vi "Main_v2.vi"() -> ()   [LabVIEW 2020]
uses:
  Shutter-DQMH/Libraries/Shutter/Shutter State.ctl
  <vilib>/Analysis/1siggen.llb/Ramp Pattern by Delta.vi
  SMC100-DQMH/Libraries/SMC100/SMC100.lvlib
  <vilib>/Analysis/NI_AALBase.lvlib
  Shutter-DQMH/Libraries/Shutter/Shutter.lvlib
panel:
  in  "CLOSED Shutter Time (s)":dbl=6.0
  in  "Fine?":bool=TRUE
  in  "Fine Steps":dbl=0.01 format="%#_6f"
  in  "Fine End":dbl=10.7
  in  "Fine Start":dbl=10.6
  out "Position":dbl=10.2
  out "Shutter State":bool
  in  "Open Shutter Panel":bool
  in  "Open Delay Stage Panel":bool
  in  "SMC100 Serial Port":u8=3
  in  "Run":bool
  out "Seconds Running":i16
  in  "OPEN Shutter Time (s)":dbl=3.0
  out "Number of Steps":i32=20
  in  "Step Size":dbl=0.09999999999999998 format="%#_6f"
  in  "End Position":dbl=11.0
  in  "Start Position":dbl=10.0
  in  "Exit":bool
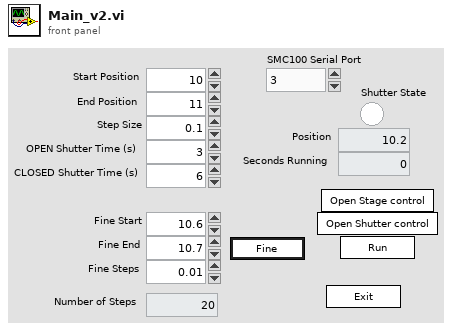
[diagram p1: front panel]
types:
  T1 = enum32{"Invalid", "Standard", "Closed", "Hidden", "Minimized", "Maximized"}
  T2 = enum32{"invalid app kind", "Development System", "Run Time System", "Student Edition", "Embedded LabVIEW", "Evaluation", "Custom"}
  T3 = typedef "Shutter State.ctl" = enum16{"None", "Open", "Closed"}
  T4 = cluster{"Core":cluster{"Current VI Reference":refnum<vi>, "Close Panel on Exit?":bool}, "Delay Positions":dbl[], "OPEN Shutter Time (s)":dbl, "Position Index":i32, "CLOSED Shutter Time (s)":dbl}
  T5 = cluster{"Current VI Reference":refnum<vi>, "Close Panel on Exit?":bool}
  T6 = typedef "SMC100.lvlib/Get Abs Position (Reply Payload)--cluster.ctl" = cluster{"Absolute Position":dbl, "Get Abs Position_error":errorcluster}
  T7 = typedef "Shutter.lvlib/Get Shutter State (Reply Payload)--cluster.ctl" = cluster{"Shutter State":T3, "Get Shutter State_error":errorcluster}
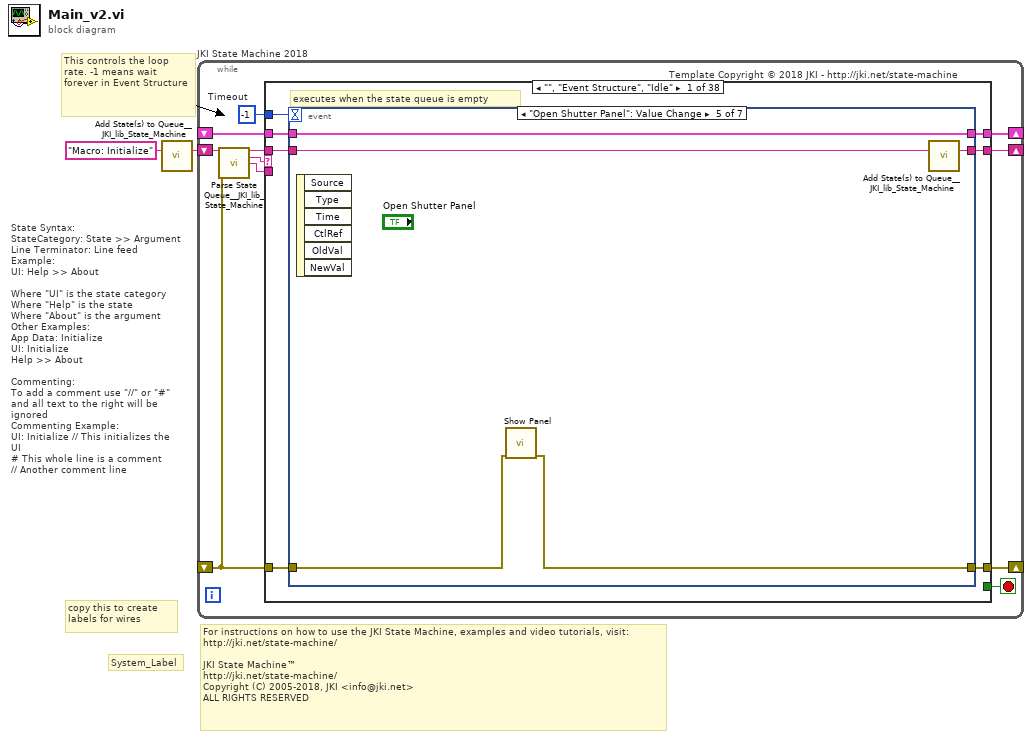
[diagram p0: block diagram]
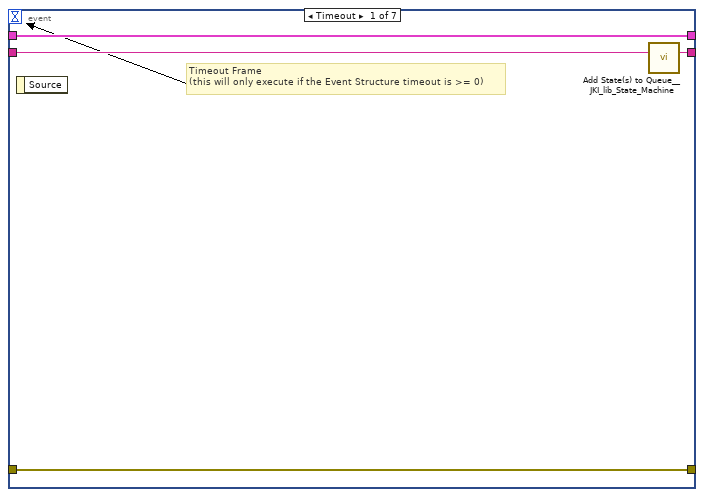
[diagram p2: hidden frame]
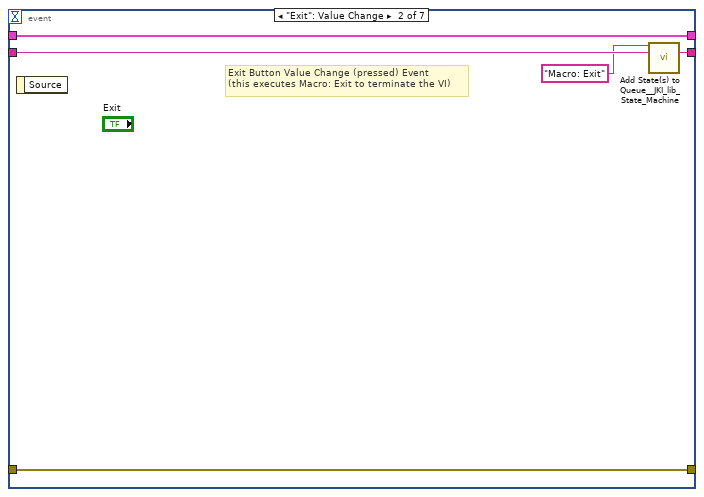
[diagram p3: hidden frame]
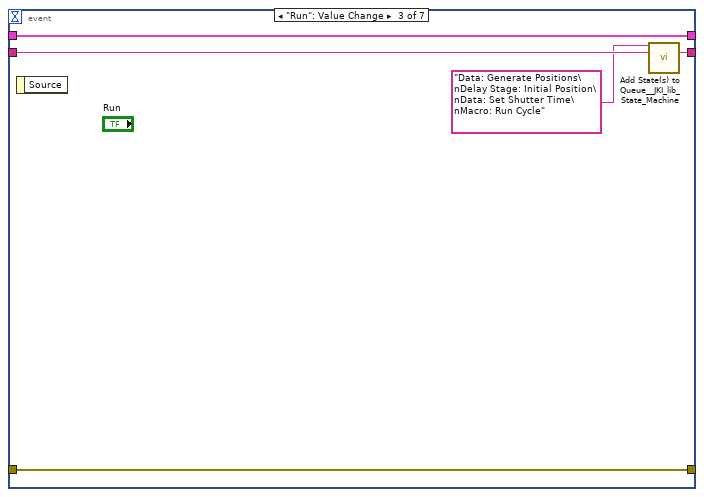
[diagram p4: hidden frame]
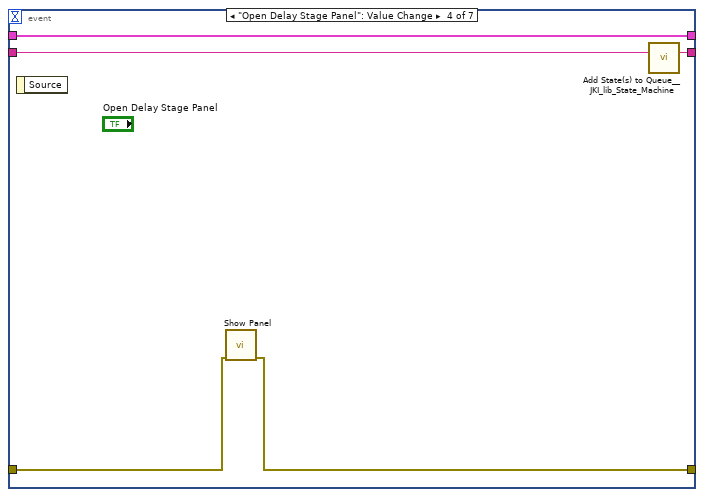
[diagram p5: hidden frame]
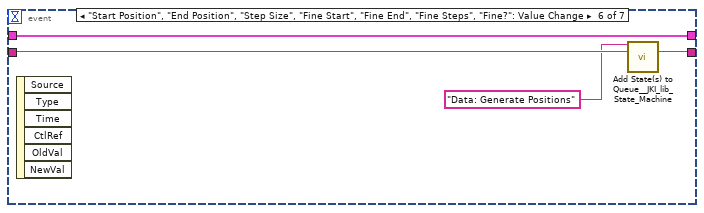
[diagram p6: hidden frame]
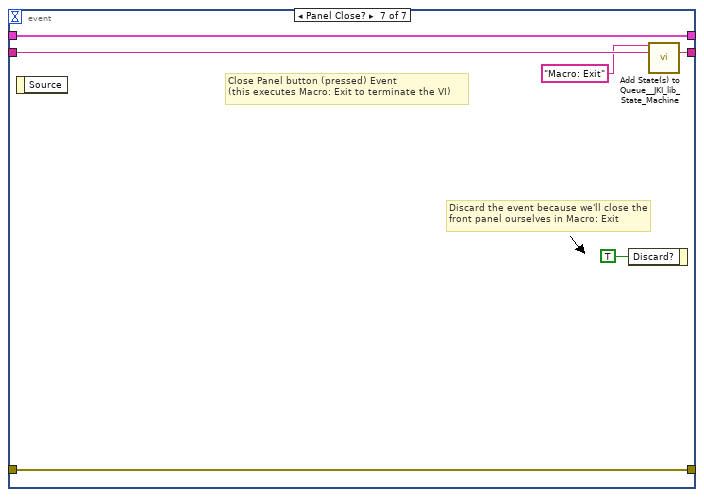
[diagram p7: hidden frame]
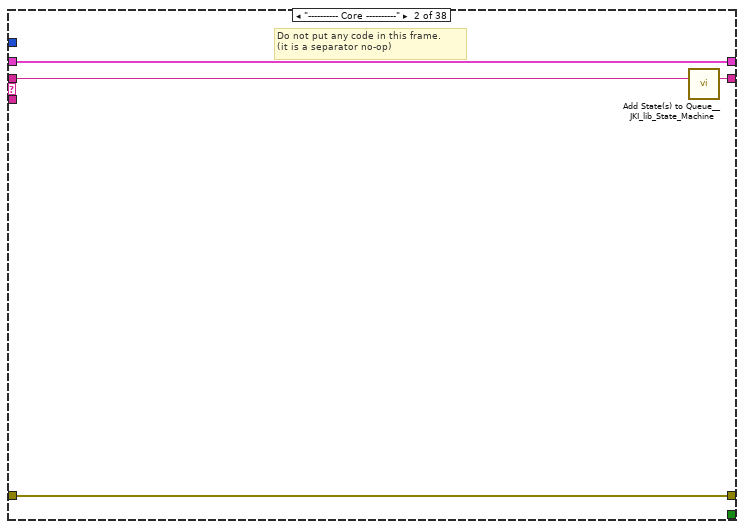
[diagram p8: hidden frame]
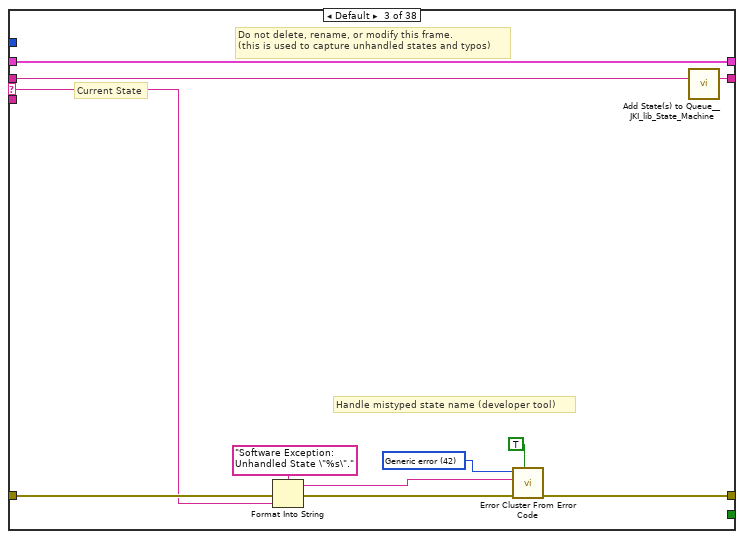
[diagram p9: hidden frame]
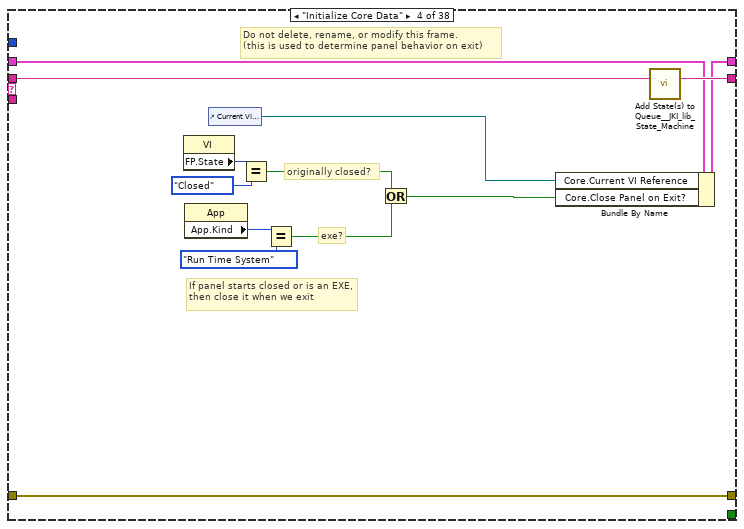
[diagram p10: hidden frame]
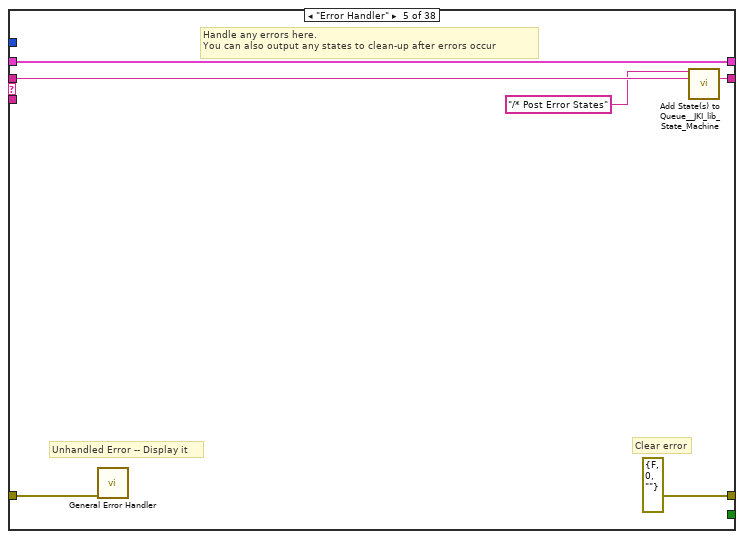
[diagram p11: hidden frame]
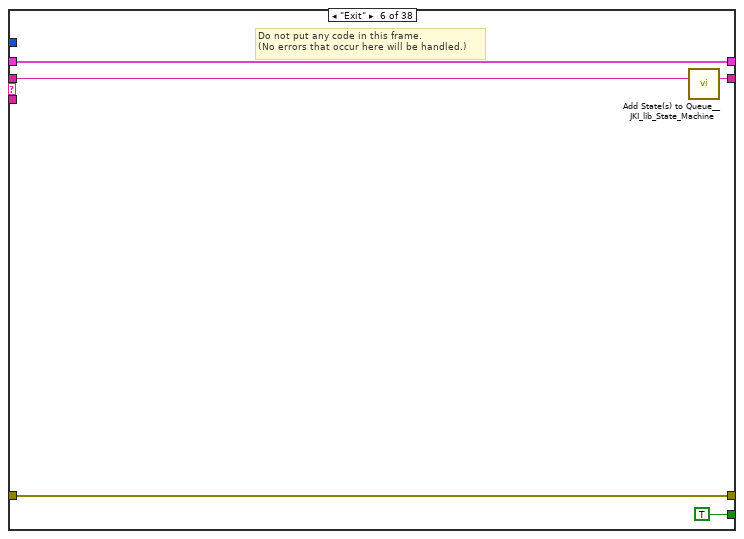
[diagram p12: hidden frame]
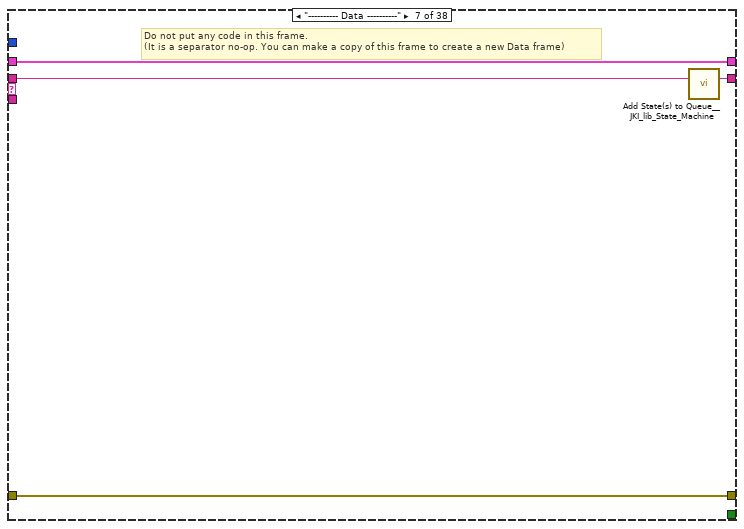
[diagram p13: hidden frame]
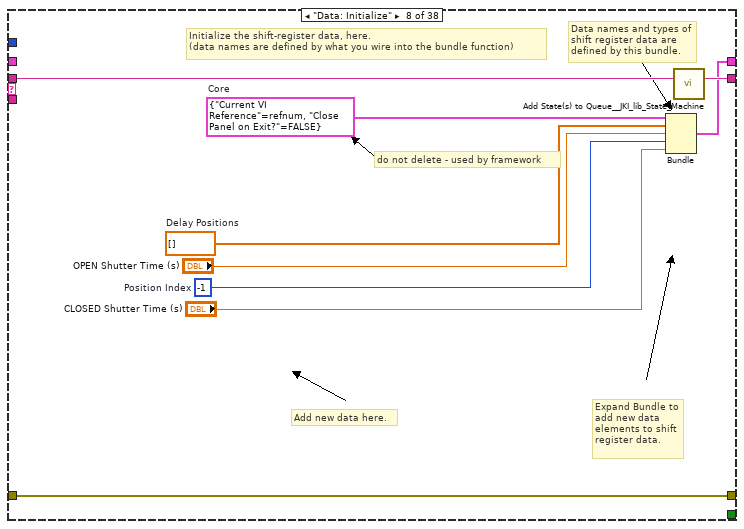
[diagram p14: hidden frame]
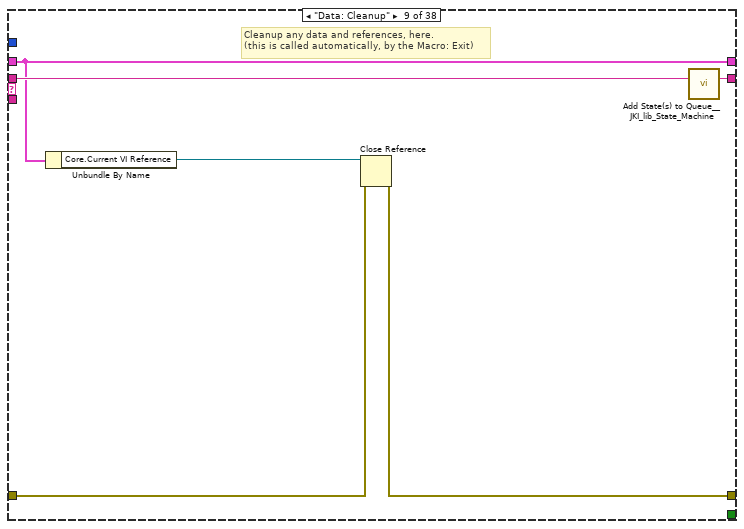
[diagram p15: hidden frame]
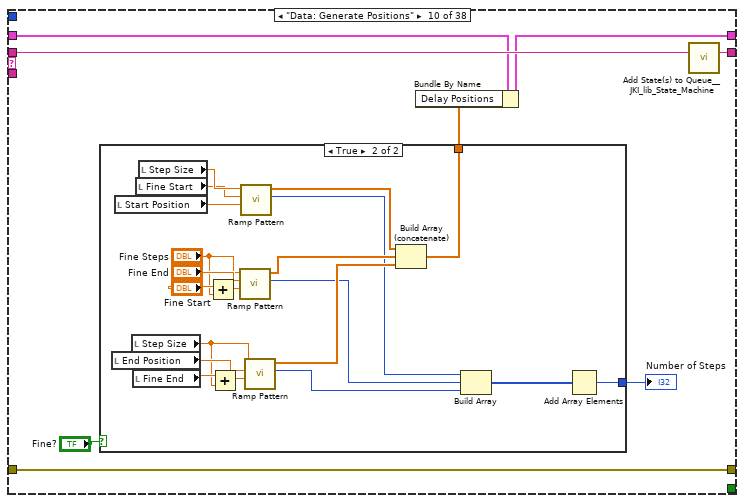
[diagram p16: hidden frame]
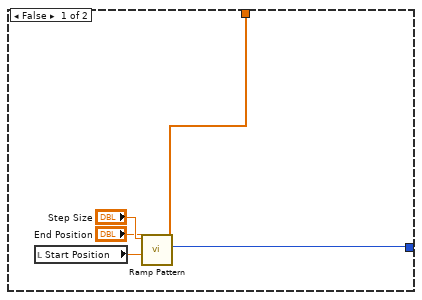
[diagram p17: hidden frame]
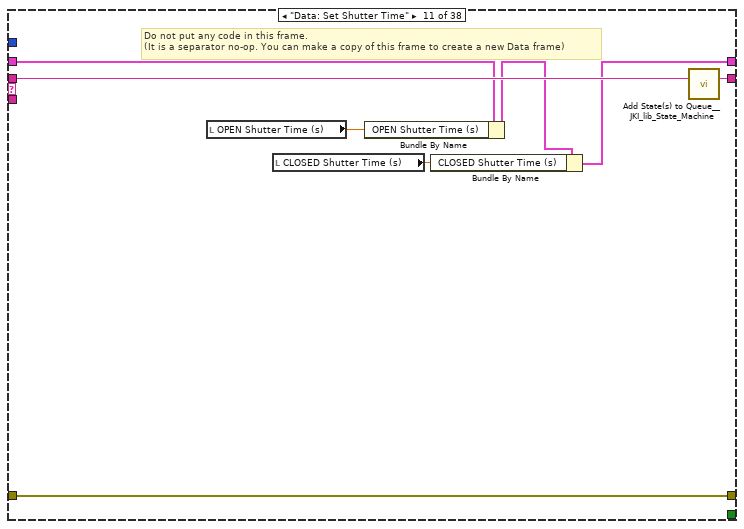
[diagram p18: hidden frame]
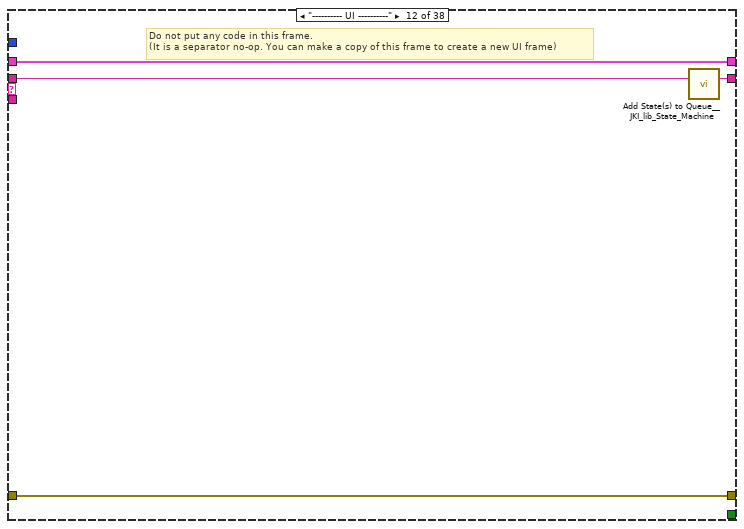
[diagram p19: hidden frame]
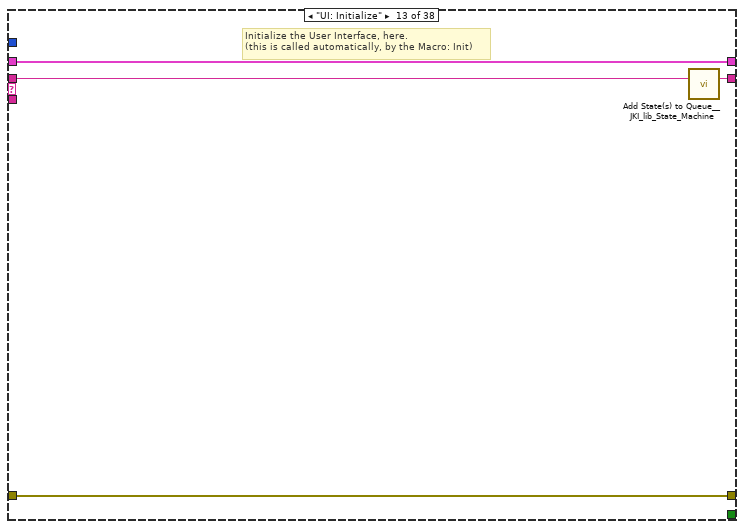
[diagram p20: hidden frame]
diagram:
  # "For instructions on how to use the JKI State Machine, examples and video tutorials, visit:\nhttp://jki.net/state-machine/\n\nJKI State Machine™\nhttp://jki.net/state-machine/\nCopyright (C) 2005-2018, JKI <info@jki.net>\nALL RIGHTS RESERVED"
  # "State Syntax:\nStateCategory: State >> Argument\nLine Terminator: Line feed\nExample:\nUI: Help >> About\n\nWhere \"UI\" is the state category\nWhere \"Help\" is the state\nWhere \"About\" is the argument\nOther Examples:\nApp Data: Initialize\nUI: Initialize\nHelp >> About\n\nCommenting:\nTo add a comment use \"//\" or \"#\" and all text to the right will be ignored\nCommenting Example:\nUI: Initialize // This initializes the UI\n# This whole line is a comment\n// Another comment line"
  # "copy this to create labels for wires"
  # "This controls the loop rate. -1 means wait forever in Event Structure"
  # "System_Label"
  n1 = call <vilib>:"Add State(s) to Queue__JKI_lib_State_Machine.vi"("State(s) in (\"\")"="Macro: Initialize") -> ("States Out"=w2:string)  [unwired: 14 in]
  n2 = while "JKI State Machine 2018" {
    shift-right: [w6] -> _
    shift-left: _ -> [w5]
    shift-right: [w9] -> _
    shift-left: _ -> [w3]
    shift-right: [w8] -> _
    shift-left: w2 -> [w10]
    stop <- w7 stop-if-true
    w4 = -1  # Timeout
    # "Template Copyright © 2018 JKI - http://jki.net/state-machine"
    n3 = call <vilib>:"Parse State Queue__JKI_lib_State_Machine.vi"("State Queue"=w10, "Error In (no error)"=w3) -> ("Remaining States"=w12:string, "Current State"=w13:string, "Arguments"=w11:string)  [unwired: 11 in]
    n4 = case shown="\"\", \"Event Structure\", \"Idle\"" w13 {
      selector: w13 -> [_ _ w59 _ _ _ _ _ _ _ _ _ _ _ _ _ _ _ _ _ _ _ _ _ _ _ _ _ _ _ _ _ _ _ _ _ _ _]
      tunnel: w12 -> [w20 w58 w63 w82 w88 w93 w97 w106 w112 w120 w153 w157 w161 w167 w178 w246 w252 w257 w262 w267 w277 w282 w286 w292 w297 w303 w314 w321 w325 w330 w335 w342 w349 w358 w362 w377 w387 w402]
      tunnel: w11 -> [_ _ _ _ _ _ _ _ _ _ _ _ _ w162 w172 _ _ _ _ _ _ _ _ _ _ _ _ _ _ _ _ _ _ _ _ _ _ _]
      tunnel: w5 -> [w18 w55 w61 w75 w85 w91 w94 _ w107 w117 w150 w154 w159 w165 w174 w245 w249 w254 w259 w264 w274 w279 w283 w289 w294 w300 w310 w318 w322 w327 w332 w339 w346 w356 w359 w374 w383 w398]
      tunnel: [w17 w56 w65 w79 errorcluster {"status"=FALSE, "code"=0, "source"=""} ("error out") w90 w95 w103 w108 w118 w151 w155 w158 w163 w175 w244 w250 w255 w260 w265 w275 w280 w284 w288 w293 w299 w311 w317 w323 w326 w331 w337 w345 w351 w360 w375 w385 w400] -> w9
      tunnel: w3 -> [w16 w56 w64 w79 w84 w90 w95 w103 w109 w118 w151 w155 w158 w164 w176 w244 w250 w255 w260 w265 w275 w280 w284 w290 w295 w301 w312 w319 w323 w328 w333 w340 w347 w352 w360 w375 w385 w400]
      tunnel: [w19 w57 w62 w81 w87 w92 w96 w105 w111 w119 w152 w156 w160 w166 w177 w247 w251 w256 w261 w266 w276 w281 w285 w291 w296 w302 w313 w320 w324 w329 w334 w341 w348 w357 w361 w376 w386 w401] -> w8
      tunnel: [_ _ _ _ _ TRUE _ _ _ _ _ _ _ _ _ _ _ _ _ _ _ _ _ _ _ _ _ _ _ _ _ _ _ _ _ _ _ _] -> w7
      tunnel: [w15 w55 w61 w80 w85 w91 w94 w104 w107 w116 w146 w154 w159 w165 w174 w245 w249 w254 w259 w264 w274 w279 w283 w289 w294 w300 w308 w318 w322 w327 w332 w339 w346 w356 w359 w370 w383 w398] -> w6
      tunnel: w4 -> [w14 _ _ _ _ _ _ _ _ _ _ _ _ _ _ _ _ _ _ _ _ _ _ _ _ _ _ _ _ _ _ _ _ _ _ _ _ _]
      frame "", "Event Structure", "Idle" {
        # "executes when the state queue is empty"
        n5 = event shown="[4] \"Open Shutter Panel\": Value Change" {
          selector: _ -> [_ _ _ _ _ _ _]
          dyn-events: _ -> [_ _ _ _ _ _ _]
          timeout: w14 -> [_ _ _ _ _ _ _]
          tunnel: w20 -> [w24 w29 w34 w39 w44 w46 w54]
          tunnel: [w23 w28 w33 w38 w43 w47 w53] -> w19
          tunnel: w18 -> [w21 w26 w31 w37 w42 w48 w51]
          tunnel: [w22 w27 w32 w36 w41 _ w52] -> w17
          tunnel: w16 -> [w22 w27 w32 w35 w40 _ w52]
          tunnel: [w21 w26 w31 w37 w42 w48 w51] -> w15
          event Timeout {
            # "Timeout Frame\n(this will only execute if the Event Structure timeout is >= 0)"
            n6 = event-data() -> ()  [unwired: 1 in, 1 out]
            n7 = call <vilib>:"Add State(s) to Queue__JKI_lib_State_Machine.vi"("State(s) in (\"\")"=w24) -> ("States Out"=w23:string)  [unwired: 14 in]
          }
          event "Exit": Value Change {
            # "Exit Button Value Change (pressed) Event\n(this executes Macro: Exit to terminate the VI)"
            n8 = event-data() -> ()  [unwired: 1 in, 1 out]
            n9 = call <vilib>:"Add State(s) to Queue__JKI_lib_State_Machine.vi"("State(s) in Front (\"\")"="Macro: Exit", "State(s) in (\"\")"=w29) -> ("States Out"=w28:string)  [unwired: 13 in]
          }
          event "Run": Value Change {
            n10 = event-data() -> ()  [unwired: 1 in, 1 out]
            n11 = call <vilib>:"Add State(s) to Queue__JKI_lib_State_Machine.vi"("State(s) in Front (\"\")"="Data: Generate Positions\nDelay Stage: Initial Position\nData: Set Shutter Time\nMacro: Run Cycle", "State(s) in (\"\")"=w34) -> ("States Out"=w33:string)  [unwired: 13 in]
          }
          event "Open Delay Stage Panel": Value Change {
            n12 = event-data() -> ()  [unwired: 1 in, 1 out]
            n13 = call "Show Panel.vi"("error in (no error)"=w35) -> ("error out"=w36:errorcluster)  [unwired: 10 in]
            n14 = call <vilib>:"Add State(s) to Queue__JKI_lib_State_Machine.vi"("State(s) in (\"\")"=w39) -> ("States Out"=w38:string)  [unwired: 14 in]
          }
          event "Open Shutter Panel": Value Change {
            n15 = event-data() -> ()  [unwired: 1 in, 6 out]
            n16 = call "Show Panel.vi"("error in (no error)"=w40) -> ("error out"=w41:errorcluster)  [unwired: 10 in]
            n17 = call <vilib>:"Add State(s) to Queue__JKI_lib_State_Machine.vi"("State(s) in (\"\")"=w44) -> ("States Out"=w43:string)  [unwired: 14 in]
          }
          event "Start Position", "End Position", "Step Size", "Fine Start", "Fine End", "Fine Steps", "Fine?": Value Change {
            n18 = event-data() -> ()  [unwired: 1 in, 6 out]
            n19 = call <vilib>:"Add State(s) to Queue__JKI_lib_State_Machine.vi"("State(s) in Front (\"\")"="Data: Generate Positions" ("State(s) in Front (\"\")"), "State(s) in (\"\")"=w46) -> ("States Out"=w47:string)  [unwired: 13 in]
          }
          event Panel Close? {
            # "Discard the event because we'll close the front panel ourselves in Macro: Exit"
            # "Close Panel button (pressed) Event\n(this executes Macro: Exit to terminate the VI)"
            n20 = event-data() -> ()  [unwired: 1 in, 1 out]
            n21 = event-data("Discard?"=TRUE) -> ()  [unwired: 1 in, 1 out]
            n22 = call <vilib>:"Add State(s) to Queue__JKI_lib_State_Machine.vi"("State(s) in Front (\"\")"="Macro: Exit", "State(s) in (\"\")"=w54) -> ("States Out"=w53:string)  [unwired: 13 in]
          }
        }
      }
      frame "---------- Core ----------" {
        # "Do not put any code in this frame.\n(it is a separator no-op)"
        n23 = call <vilib>:"Add State(s) to Queue__JKI_lib_State_Machine.vi"("State(s) in (\"\")"=w58) -> ("States Out"=w57:string)  [unwired: 14 in]
      }
      frame Default {
        w68 = 42 items=["No error", "Argument error", "Memory is full", "Out of zone", "End of file", "File already open", "Generic file I/O error", "File not found", "File permission error", "Disk is full", "Duplicate path", "Too many files open", "System feature not enabled", "Resource file not found", "Cannot add resource", "Resource not found", "Image not found", "Image memory error", "Pen does not exist", "Config type invalid", "Config token not found", "Config parse error", "Config memory error", "Bad external code format", "Bad external code offset", "External code not present", "Null window", "Destroy window error", "Null menu", "Print aborted", "Bad print record", "Print driver error", "Windows error during printing", "Memory error during printing", "Print dialog error", "Generic print error", "Invalid device refnum", "Device not found", "Device parameter error", "Device unit error", "Cannot open device", "Device call aborted", "Generic error", "Cancelled by user", "Object ID too low", "Object ID too high", "Object not in heap", "Unknown heap", "Unknown object (invalid DefProc)", "Unknown object (DefProc not in table)", "Message out of range", "Invalid (null) method", "Unknown message", "Manager call not supported", "Bad address", "Network operation in progress", "Network operation timed out", "Connection is busy", "Network attribute not supported", "Network error", "Address in use", "System out of memory", "Connection aborted", "Connection refused", "Not connected", "Already connected", "Connection closed", "Initialization error (interapplication manager)", "Bad occurrence", "Wait on unbound occurrence handler", "Occurrence queue overflow", "Datalog type conflict", "Unused", "Unrecognized type (interapplication manager)", "Memory corrupt", "Failed to make temporary DLL", "Old CIN version", "Drag socket not found", "Failed to load drop-object", "Failed to register OLE object", "Failed to release OLE object", "Format specifier type mismatch", "Unknown format specifier", "Too few format specifiers", "Too many format specifiers", "Scan failed", "Newer CIN version", "Error converting to variant", "Runtime menu error", "Password tampered", "Variant attribute not found", "Incompatible variant data type", "Event data is not available", "Event Store is not present", "Occurrence is not found", "Event Queue is not created", "Event info is not available", "Refnum passed is NULL", "Error retrieving Class GUID", "Error retrieving CoClass GUID", "Error retrieving TypeLib GUID.", "Bad built application magic bytes.", "Specific driver is different from the specific driver associated with the Logical Name.", "There is no session opened to the class driver.", "Max Error", "MAX - Error with config objects", "MAX - Error loading configuration", "MAX - Group not supported"]
        # "Current State"
        # "Do not delete, rename, or modify this frame.\n(this is used to capture unhandled states and typos)"
        # "Handle mistyped state name (developer tool)"
        n24 = Format Into String(format string="Software Exception: Unhandled State \"%s\"." ("message"), error in=w64, w59) -> (resulting string=w67:string, error out=w66:errorcluster)  [unwired: 1 in]
        n25 = call <vilib>:"Error Cluster From Error Code.vi"("show call chain? (False)"=TRUE, "error in (no error)"=w66, "error message (\"\")"=w67, "error code (0)"=w68) -> ("error out"=w65:errorcluster)  [unwired: 5 in]
        n26 = call <vilib>:"Add State(s) to Queue__JKI_lib_State_Machine.vi"("State(s) in (\"\")"=w63) -> ("States Out"=w62:string)  [unwired: 14 in]
      }
      frame "Initialize Core Data" {
        # "Do not delete, rename, or modify this frame.\n(this is used to determine panel behavior on exit)"
        # "originally closed?"
        # "exe?"
        # "If panel starts closed or is an EXE, then close it when we exit"
        n27 = property class="VI"() -> ("FP.State"=w72:T1)  [unwired: 2 in, 2 out]
        n28 = property class="App"() -> ("App.Kind"=w78:T2)  [unwired: 2 in, 2 out]
        n29 = control-ref of="Current VI Reference"() -> (w73:refnum<vi>)
        n30 = Equal?(x=w72, y=T1."Closed" ("Front Panel Window:State")) -> (x = y?=w70:bool)
        n31 = Equal?(x=w78, y=T2."Run Time System" ("Application:Kind")) -> (x = y?=w76:bool)
        n32 = Or(x=w70, y=w76) -> (x .or. y?=w74:bool)
        n33 = Bundle By Name(cluster=w75, "Core.Current VI Reference"=w73, "Core.Close Panel on Exit?"=w74) -> (w80:T4)
        n34 = call <vilib>:"Add State(s) to Queue__JKI_lib_State_Machine.vi"("State(s) in (\"\")"=w82) -> ("States Out"=w81:string)  [unwired: 14 in]
      }
      frame "Error Handler" {
        # "Unhandled Error -- Display it"
        # "Handle any errors here.\nYou can also output any states to clean-up after errors occur"
        # "Clear error"
        n35 = call <vilib>:"General Error Handler.vi"("error in (no error)"=w84) -> ()  [unwired: 10 in, 5 out]
        n36 = call <vilib>:"Add State(s) to Queue__JKI_lib_State_Machine.vi"("State(s) in Front (\"\")"="/* Post Error States", "State(s) in (\"\")"=w88) -> ("States Out"=w87:string)  [unwired: 13 in]
      }
      frame "Exit" {
        # "Do not put any code in this frame.\n(No errors that occur here will be handled.)"
        n37 = call <vilib>:"Add State(s) to Queue__JKI_lib_State_Machine.vi"("State(s) in (\"\")"=w93) -> ("States Out"=w92:string)  [unwired: 14 in]
      }
      frame "---------- Data ----------" {
        # "Do not put any code in this frame.\n(It is a separator no-op. You can make a copy of this frame to create a new Data frame)"
        n38 = call <vilib>:"Add State(s) to Queue__JKI_lib_State_Machine.vi"("State(s) in (\"\")"=w97) -> ("States Out"=w96:string)  [unwired: 14 in]
      }
      frame "Data: Initialize" {
        w100 = -1  # Position Index
        w101 = dbl[] []  # Delay Positions
        w102 = T5 {"Current VI Reference"=refnum, "Close Panel on Exit?"=FALSE}  # Core
        # "do not delete - used by framework"
        # "Expand Bundle to add new data elements to shift register data."
        # "Add new data here."
        # "Data names and types of shift register data are defined by this bundle."
        # "Initialize the shift-register data, here.\n(data names are defined by what you wire into the bundle function)"
        n39 = Bundle("Core"=w102, "Delay Positions"=w101, "OPEN Shutter Time (s)"="OPEN Shutter Time (s)", "Position Index"=w100, "CLOSED Shutter Time (s)"="CLOSED Shutter Time (s)") -> (w104:T4)  [unwired: 1 in]
        n40 = call <vilib>:"Add State(s) to Queue__JKI_lib_State_Machine.vi"("State(s) in (\"\")"=w106) -> ("States Out"=w105:string)  [unwired: 14 in]
      }
      frame "Data: Cleanup" {
        # "Cleanup any data and references, here.\n(this is called automatically, by the Macro: Exit)"
        n41 = Unbundle By Name(w107) -> ("Core.Current VI Reference"=w110:refnum<vi>)
        n42 = Close Reference(reference=w110, error in (no error)=w109) -> (error out=w108:errorcluster)
        n43 = call <vilib>:"Add State(s) to Queue__JKI_lib_State_Machine.vi"("State(s) in (\"\")"=w112) -> ("States Out"=w111:string)  [unwired: 14 in]
      }
      frame "Data: Generate Positions" {
        n44 = case shown="True" "Fine?" {
          tunnel: [w122 w127] -> w114
          tunnel: [w121 w126] -> w113
          frame False {
            n45 = local read "Start Position"() -> (w123:dbl)
            n46 = call-poly <vilib>:"Ramp Pattern.vi"("start"=w123, "end"="End Position", "delta"="Step Size") -> ("samples"=w122:i32, "Ramp Pattern"=w121:dbl[])  [unwired: 6 in, 1 out]
          }
          frame True {
            n47 = local read "End Position"() -> (w138:dbl)
            n48 = local read "Start Position"() -> (w143:dbl)
            n49 = local read "Step Size"() -> (w135:dbl)
            n50 = local read "Fine End"() -> (w137:dbl)
            n51 = local read "Fine Start"() -> (w141:dbl)
            n52 = local read "Step Size"() -> (w142:dbl)
            n53 = Add(x="Fine Start", y="Fine Steps") -> (x+y=w140:dbl)
            n54 = Add(x=w137, y=w135) -> (x+y=w136:dbl)
            n55 = call-poly <vilib>:"Ramp Pattern.vi"("start"=w140, "end"="Fine End", "delta"="Fine Steps") -> ("samples"=w130:i32, "Ramp Pattern"=w133:dbl[])  [unwired: 6 in, 1 out]
            n56 = call-poly <vilib>:"Ramp Pattern.vi"("start"=w143, "end"=w141, "delta"=w142) -> ("samples"=w129:i32, "Ramp Pattern"=w134:dbl[])  [unwired: 6 in, 1 out]
            n57 = call-poly <vilib>:"Ramp Pattern.vi"("start"=w136, "end"=w138, "delta"=w135) -> ("samples"=w131:i32, "Ramp Pattern"=w132:dbl[])  [unwired: 6 in, 1 out]
            n58 = Build Array (concatenate)(w134, w133, w132) -> (w126:dbl[])
            n59 = Build Array(w129, w130, w131) -> (w128:i32[])
            n60 = Add Array Elements(numeric array=w128) -> (sum=w127:i32)
          }
        }
        "Number of Steps" <- w114
        n61 = Bundle By Name(cluster=w117, "Delay Positions"=w113) -> (w116:T4)
        n62 = call <vilib>:"Add State(s) to Queue__JKI_lib_State_Machine.vi"("State(s) in (\"\")"=w120) -> ("States Out"=w119:string)  [unwired: 14 in]
      }
      frame "Data: Set Shutter Time" {
        # "Do not put any code in this frame.\n(It is a separator no-op. You can make a copy of this frame to create a new Data frame)"
        n63 = local read "OPEN Shutter Time (s)"() -> (w149:dbl)
        n64 = local read "CLOSED Shutter Time (s)"() -> (w148:dbl)
        n65 = Bundle By Name(cluster=w150, "OPEN Shutter Time (s)"=w149) -> (w147:T4)
        n66 = Bundle By Name(cluster=w147, "CLOSED Shutter Time (s)"=w148) -> (w146:T4)
        n67 = call <vilib>:"Add State(s) to Queue__JKI_lib_State_Machine.vi"("State(s) in (\"\")"=w153) -> ("States Out"=w152:string)  [unwired: 14 in]
      }
      frame "---------- UI ----------" {
        # "Do not put any code in this frame.\n(It is a separator no-op. You can make a copy of this frame to create a new UI frame)"
        n68 = call <vilib>:"Add State(s) to Queue__JKI_lib_State_Machine.vi"("State(s) in (\"\")"=w157) -> ("States Out"=w156:string)  [unwired: 14 in]
      }
      frame "UI: Initialize" {
        # "Initialize the User Interface, here.\n(this is called automatically, by the Macro: Init)"
        n69 = call <vilib>:"Add State(s) to Queue__JKI_lib_State_Machine.vi"("State(s) in (\"\")"=w161) -> ("States Out"=w160:string)  [unwired: 14 in]
      }
      frame "UI: Cursor Set" {
        # "Argument"
        # "Set and Unset Cursor Busy.\n(Usage: \"UI: Cursor Set >> Busy|Idle\")"
        n70 = case shown="\"Idle\", Default" w162 {
          tunnel: w164 -> [w169 w171]
          tunnel: [w168 w170] -> w163
          frame "Idle", Default {
            n71 = call <vilib>:"Unset Busy.vi"("error in (no error)"=w169) -> ("error out"=w168:errorcluster)  [unwired: 10 in]
          }
          frame "Busy" {
            n72 = call <vilib>:"Set Busy.vi"("error in (no error)"=w171) -> ("error out"=w170:errorcluster)  [unwired: 9 in, 1 out]
          }
        }
        n73 = call <vilib>:"Add State(s) to Queue__JKI_lib_State_Machine.vi"("State(s) in (\"\")"=w167) -> ("States Out"=w166:string)  [unwired: 14 in]
      }
      frame "UI: Front Panel State" {
        # "Argument"
        # "Set Front Panel Open or Closed\n(Usage: \"UI: Front Panel State >> Open|Close\")"
        n74 = Unbundle By Name(w174) -> ("Core.Current VI Reference"=w173:refnum<vi>)
        n75 = case shown="\"Minimize\", \"Minimized\"" w172 {
          tunnel: w176 -> [w184 w199 w210 w223 w236]
          tunnel: [w186 w200 w212 w225 w238] -> w175
          tunnel: w173 -> [w185 w197 w211 w224 w237]
          frame "Open", "Standard", Default {
            w179 = T1."Standard" ("State")
            n76 = property class="VI"(reference=w185, error in=w184) -> (reference out=w182:refnum<vi>, error out=w183:errorcluster, "FP.State"=w181:T1)
            n77 = Not Equal?(x=w181, y=w179) -> (x != y?=w180:bool)
            n78 = case shown="True" w180 {
              tunnel: [w190 w192] -> w186
              tunnel: w183 -> [w189 w192]
              tunnel: w182 -> [w188 _]
              tunnel: w179 -> [w187 _]
              frame True {
                n79 = invoke class="VI" method="FP.Open"(reference=w188, error in=w189, "Activate"=TRUE, "State"=w187) -> (error out=w190:errorcluster)  [unwired: 1 in, 4 out]
              }
              frame False {
              }
            }
          }
          frame "Close", "Closed" {
            n80 = property class="VI"(reference=w197, error in=w199) -> (reference out=w196:refnum<vi>, error out=w198:errorcluster, "FP.State"=w194:T1)
            n81 = Not Equal?(x=w194, y=T1."Closed" ("Front Panel Window:State")) -> (x != y?=w193:bool)
            n82 = case shown="True" w193 {
              tunnel: [w201 w204] -> w200
              tunnel: w198 -> [w201 w203]
              tunnel: w196 -> [_ w202]
              frame False {
              }
              frame True {
                n83 = invoke class="VI" method="FP.Close"(reference=w202, error in=w203) -> (error out=w204:errorcluster)  [unwired: 1 in, 2 out]
              }
            }
          }
          frame "Hidden", "Hide" {
            w205 = T1."Hidden" ("State")
            n84 = property class="VI"(reference=w211, error in=w210) -> (reference out=w208:refnum<vi>, error out=w209:errorcluster, "FP.State"=w207:T1)
            n85 = Not Equal?(x=w207, y=w205) -> (x != y?=w206:bool)
            n86 = case shown="True" w206 {
              tunnel: [w216 w217] -> w212
              tunnel: w209 -> [w215 w217]
              tunnel: w208 -> [w214 _]
              tunnel: w205 -> [w213 _]
              frame True {
                n87 = invoke class="VI" method="FP.Open"(reference=w214, error in=w215, "State"=w213) -> (error out=w216:errorcluster)  [unwired: 2 in, 4 out]
              }
              frame False {
              }
            }
          }
          frame "Minimize", "Minimized" {
            w218 = T1."Minimized" ("State")
            n88 = property class="VI"(reference=w224, error in=w223) -> (reference out=w221:refnum<vi>, error out=w222:errorcluster, "FP.State"=w220:T1)
            n89 = Not Equal?(x=w220, y=w218) -> (x != y?=w219:bool)
            n90 = case shown="True" w219 {
              tunnel: [w229 w230] -> w225
              tunnel: w222 -> [w228 w230]
              tunnel: w221 -> [w227 _]
              tunnel: w218 -> [w226 _]
              frame True {
                n91 = invoke class="VI" method="FP.Open"(reference=w227, error in=w228, "State"=w226) -> (error out=w229:errorcluster)  [unwired: 2 in, 4 out]
              }
              frame False {
              }
            }
          }
          frame "Maximize", "Maximized" {
            w231 = T1."Maximized" ("State")
            n92 = property class="VI"(reference=w237, error in=w236) -> (reference out=w234:refnum<vi>, error out=w235:errorcluster, "FP.State"=w233:T1)
            n93 = Not Equal?(x=w233, y=w231) -> (x != y?=w232:bool)
            n94 = case shown="True" w232 {
              tunnel: [w242 w243] -> w238
              tunnel: w235 -> [w241 w243]
              tunnel: w234 -> [w240 _]
              tunnel: w231 -> [w239 _]
              frame True {
                n95 = invoke class="VI" method="FP.Open"(reference=w240, error in=w241, "State"=w239) -> (error out=w242:errorcluster)  [unwired: 2 in, 4 out]
              }
              frame False {
              }
            }
          }
        }
        n96 = call <vilib>:"Add State(s) to Queue__JKI_lib_State_Machine.vi"("State(s) in (\"\")"=w178) -> ("States Out"=w177:string)  [unwired: 14 in]
      }
      frame "UI: Stop Exit" {
        n97 = local write "Exit"(FALSE ("Run")) -> ()
        n98 = call <vilib>:"Add State(s) to Queue__JKI_lib_State_Machine.vi"("State(s) in (\"\")"=w246) -> ("States Out"=w247:string)  [unwired: 14 in]
      }
      frame "---------- Macro ----------" {
        # "Do not put any code in this frame.\n(It is a separator no-op. You can make a copy of this frame to create a new Macro frame)"
        n99 = call <vilib>:"Add State(s) to Queue__JKI_lib_State_Machine.vi"("State(s) in (\"\")"=w252) -> ("States Out"=w251:string)  [unwired: 14 in]
      }
      frame "Macro: Run Cycle" {
        n100 = call <vilib>:"Add State(s) to Queue__JKI_lib_State_Machine.vi"("State(s) in Front (\"\")"="Shutter: Close\nShutter: Get Shutter State\nDelay Stage: Move Next\nDelay Stage: Get Position\nHelpers: Wait Closed\nShutter: Open\nShutter: Get Shutter State\nHelpers: Wait\nHelpers: At End?" ("State(s) in Front (\"\")"), "State(s) in (\"\")"=w257) -> ("States Out"=w256:string)  [unwired: 13 in]
      }
      frame "Macro: Initialize" {
        # "Initialization Macro\n(This is called once, when the VI starts)"
        n101 = call <vilib>:"Add State(s) to Queue__JKI_lib_State_Machine.vi"("State(s) in Front (\"\")"="Data: Initialize\nInitialize Core Data\nDelay Stage: Start Module\nShutter: Start Module\nUI: Initialize\nUI: Front Panel State >> Open\nUI: Stop Exit", "State(s) in (\"\")"=w262) -> ("States Out"=w261:string)  [unwired: 13 in]
      }
      frame "Macro: Initial Device States" {
        n102 = call <vilib>:"Add State(s) to Queue__JKI_lib_State_Machine.vi"("State(s) in Front (\"\")"="Delay Stage: Initial Position" ("State(s) in Front (\"\")"), "State(s) in (\"\")"=w267) -> ("States Out"=w266:string)  [unwired: 13 in]
      }
      frame "Macro: Exit" {
        # "Exit Macro\n(This is called once, when the VI exits)"
        n103 = Unbundle By Name(w274) -> ("Core.Close Panel on Exit?"=w273:bool)
        n104 = Select(t="UI: Front Panel State >> Close", s=w273, f="") -> (s? t:f=w270:string)
        n105 = call <vilib>:"Add State(s) to Queue__JKI_lib_State_Machine.vi"("State(s) in (\"\")"=w270, "State(s) at Back (\"\")"="Delay Stage: Stop Module\nShutter: Stop Module\nData: Cleanup\nExit") -> ("States Out"=w268:string)  [unwired: 13 in]
        n106 = call <vilib>:"Add State(s) to Queue__JKI_lib_State_Machine.vi"("State(s) in Front (\"\")"=w268, "State(s) in (\"\")"=w277) -> ("States Out"=w276:string)  [unwired: 13 in]
      }
      frame "Macro: Device Cleanup" {
        # "Do not put any code in this frame.\n(It is a separator no-op. You can make a copy of this frame to create a new Macro frame)"
        n107 = call <vilib>:"Add State(s) to Queue__JKI_lib_State_Machine.vi"("State(s) in Front (\"\")"="Shutter: Close\nShutter: Get Shutter State\nDelay Stage: Get Position\nUI: Stop Exit" ("State(s) in Front (\"\")"), "State(s) in (\"\")"=w282) -> ("States Out"=w281:string)  [unwired: 13 in]
      }
      frame "---------- Delay Stage ----------" {
        # "Template Separator\n(You can make a copy of, or modify, this frame)"
        n108 = call <vilib>:"Add State(s) to Queue__JKI_lib_State_Machine.vi"("State(s) in (\"\")"=w286) -> ("States Out"=w285:string)  [unwired: 14 in]
      }
      frame "Delay Stage: Start Module" {
        # "Template Separator\n(You can make a copy of, or modify, this frame)"
        n109 = call "Start Module.vi"("error in (no error)"=w290, "SerialPort"="SMC100 Serial Port") -> ("error out"=w288:errorcluster)  [unwired: 6 in, 3 out]
        n110 = call <vilib>:"Add State(s) to Queue__JKI_lib_State_Machine.vi"("State(s) in (\"\")"=w292) -> ("States Out"=w291:string)  [unwired: 14 in]
      }
      frame "Delay Stage: Stop Module" {
        # "Template Separator\n(You can make a copy of, or modify, this frame)"
        n111 = call "Stop Module.vi"("error in (no error)"=w295) -> ("error out"=w293:errorcluster)  [unwired: 10 in]
        n112 = call <vilib>:"Add State(s) to Queue__JKI_lib_State_Machine.vi"("State(s) in (\"\")"=w297) -> ("States Out"=w296:string)  [unwired: 14 in]
      }
      frame "Delay Stage: Initial Position" {
        # "Your code here.\n(You can make a copy of, or modify, this frame)"
        n113 = call "Set Abs Position.vi"("error in (no error)"=w301, "Abolute Position"="Start Position") -> ("error out"=w299:errorcluster)  [unwired: 9 in]
        n114 = call <vilib>:"Add State(s) to Queue__JKI_lib_State_Machine.vi"("State(s) in (\"\")"=w303) -> ("States Out"=w302:string)  [unwired: 14 in]
      }
      frame "Delay Stage: Move Next" {
        # "Your code here.\n(You can make a copy of, or modify, this frame)"
        n115 = Unbundle By Name(w310) -> ("Delay Positions"=w309:dbl[], "Position Index"=w307:i32)
        n116 = Increment(x=w307) -> (x+1=w306:i32)
        n117 = Bundle By Name(cluster=w310, "Position Index"=w306) -> (w308:T4)
        n118 = Index Array(array=w309, index=w306) -> (element=w305:dbl)
        n119 = call "Set Abs Position.vi"("error in (no error)"=w312, "Abolute Position"=w305) -> ("error out"=w311:errorcluster)  [unwired: 9 in]
        n120 = Wait (ms)(milliseconds to wait=u32 1000) -> ()  [unwired: 1 out]
        n121 = call <vilib>:"Add State(s) to Queue__JKI_lib_State_Machine.vi"("State(s) in (\"\")"=w314) -> ("States Out"=w313:string)  [unwired: 14 in]
      }
      frame "Delay Stage: Get Position" {
        # "Template Separator\n(You can make a copy of, or modify, this frame)"
        n122 = call "Get Abs Position.vi"("error in (no error)"=w319) -> ("error out"=w317:errorcluster, "Reply Payload"=w316:T6)  [unwired: 8 in, 1 out]
        n123 = Unbundle By Name(w316) -> ("Absolute Position"=→"Position":dbl)
        n124 = call <vilib>:"Add State(s) to Queue__JKI_lib_State_Machine.vi"("State(s) in (\"\")"=w321) -> ("States Out"=w320:string)  [unwired: 14 in]
      }
      frame "---------- Shutter ----------" {
        # "Your code here.\n(You can make a copy of, or modify, this frame)"
        n125 = call <vilib>:"Add State(s) to Queue__JKI_lib_State_Machine.vi"("State(s) in (\"\")"=w325) -> ("States Out"=w324:string)  [unwired: 14 in]
      }
      frame "Shutter: Start Module" {
        # "Your code here.\n(You can make a copy of, or modify, this frame)"
        n126 = call "Start Module.vi"("error in (no error)"=w328) -> ("error out"=w326:errorcluster)  [unwired: 7 in, 3 out]
        n127 = call <vilib>:"Add State(s) to Queue__JKI_lib_State_Machine.vi"("State(s) in (\"\")"=w330) -> ("States Out"=w329:string)  [unwired: 14 in]
      }
      frame "Shutter: Stop Module" {
        # "Your code here.\n(You can make a copy of, or modify, this frame)"
        n128 = call "Stop Module.vi"("error in (no error)"=w333) -> ("error out"=w331:errorcluster)  [unwired: 10 in]
        n129 = call <vilib>:"Add State(s) to Queue__JKI_lib_State_Machine.vi"("State(s) in (\"\")"=w335) -> ("States Out"=w334:string)  [unwired: 14 in]
      }
      frame "Shutter: Open" {
        # "Your code here.\n(You can make a copy of, or modify, this frame)"
        n130 = call "Set Shutter State.vi"("error in (no error)"=w340, "Shutter State"=Shutter_State."Open") -> ("error out"=w337:errorcluster)  [unwired: 7 in, 2 out]
        n131 = Wait (ms)(milliseconds to wait=u32 200) -> ()  [unwired: 1 out]
        n132 = call <vilib>:"Add State(s) to Queue__JKI_lib_State_Machine.vi"("State(s) in (\"\")"=w342) -> ("States Out"=w341:string)  [unwired: 14 in]
      }
      frame "Shutter: Close" {
        # "Your code here.\n(You can make a copy of, or modify, this frame)"
        n133 = call "Set Shutter State.vi"("error in (no error)"=w347, "Shutter State"=Shutter_State."Closed") -> ("error out"=w345:errorcluster)  [unwired: 7 in, 2 out]
        n134 = Wait (ms)(milliseconds to wait=u32 200) -> ()  [unwired: 1 out]
        n135 = call <vilib>:"Add State(s) to Queue__JKI_lib_State_Machine.vi"("State(s) in (\"\")"=w349) -> ("States Out"=w348:string)  [unwired: 14 in]
      }
      frame "Shutter: Get Shutter State" {
        # "Your code here.\n(You can make a copy of, or modify, this frame)"
        n136 = call "Get Shutter State.vi"("error in (no error)"=w352) -> ("error out"=w351:errorcluster, "Reply Payload"=w355:T7)  [unwired: 8 in, 1 out]
        n137 = Unbundle By Name(w355) -> ("Shutter State"=w354:T3)
        n138 = Equal?(x=Shutter_State."Open" ("Shutter State"), y=w354) -> (x = y?=→"Shutter State":bool)
        n139 = call <vilib>:"Add State(s) to Queue__JKI_lib_State_Machine.vi"("State(s) in (\"\")"=w358) -> ("States Out"=w357:string)  [unwired: 14 in]
      }
      frame "---------- Helpers ----------" {
        # "Your code here.\n(You can make a copy of, or modify, this frame)"
        n140 = call <vilib>:"Add State(s) to Queue__JKI_lib_State_Machine.vi"("State(s) in (\"\")"=w362) -> ("States Out"=w361:string)  [unwired: 14 in]
      }
      frame "Helpers: At End?" {
        # "Your code here.\n(You can make a copy of, or modify, this frame)"
        n141 = Unbundle By Name(w374) -> ("Position Index"=w367:i32, "Delay Positions"=w369:dbl[])
        n142 = Increment(x=w367) -> (x+1=w366:i32)
        n143 = Array Size(array=w369) -> (size(s)=w368:i32)
        n144 = Greater Or Equal?(x=w366, y=w368) -> (x >= y?=w365:bool)
        n145 = local read "Exit"() -> (w363:bool)
        n146 = Or(x=w363, y=w365) -> (x .or. y?=w364:bool)
        n147 = Select(t="Macro: Device Cleanup", s=w364, f="Macro: Run Cycle") -> (s? t:f=w371:string)
        n148 = case shown="True" w364 {
          tunnel: w374 -> [w378 w381]
          tunnel: [w378 w380] -> w370
          frame False {
          }
          frame True {
            n149 = Bundle By Name(cluster=w381, "Position Index"=0) -> (w380:T4)
          }
        }
        n150 = call <vilib>:"Add State(s) to Queue__JKI_lib_State_Machine.vi"("State(s) in Front (\"\")"=w371, "State(s) in (\"\")"=w377) -> ("States Out"=w376:string)  [unwired: 13 in]
      }
      frame "Helpers: Wait" {
        # "Your code here.\n(You can make a copy of, or modify, this frame)"
        n151 = Unbundle By Name(w383) -> ("OPEN Shutter Time (s)"=w382:dbl)
        n152 = Tick Count (ms)() -> (millisecond timer value=w384:u32)
        n153 = while {
          tunnel: w384 -> [w395]
          tunnel: w382 -> [w393]
          stop <- w389 stop-if-true
          n154 = Tick Count (ms)() -> (millisecond timer value=w396:u32)
          n155 = Subtract(x=w396, y=w395) -> (x-y=w394:u32)
          n156 = Divide(x=w394, y=u32 1000) -> (x/y=w390:dbl)
          "Seconds Running" <- w390
          n157 = local read "Exit"() -> (w388:bool)
          n158 = Greater Or Equal?(x=w390, y=w393) -> (x >= y?=w391:bool)
          n159 = Or(x=w391, y=w388) -> (x .or. y?=w389:bool)
        }
        n160 = call <vilib>:"Add State(s) to Queue__JKI_lib_State_Machine.vi"("State(s) in (\"\")"=w387) -> ("States Out"=w386:string)  [unwired: 14 in]
      }
      frame "Helpers: Wait Closed" {
        # "Your code here.\n(You can make a copy of, or modify, this frame)"
        n161 = Unbundle By Name(w398) -> ("CLOSED Shutter Time (s)"=w397:dbl)
        n162 = Tick Count (ms)() -> (millisecond timer value=w399:u32)
        n163 = while {
          tunnel: w399 -> [w410]
          tunnel: w397 -> [w408]
          stop <- w405 stop-if-true
          n164 = Tick Count (ms)() -> (millisecond timer value=w411:u32)
          n165 = Subtract(x=w411, y=w410) -> (x-y=w409:u32)
          n166 = Divide(x=w409, y=u32 1000) -> (x/y=w403:dbl)
          n167 = local write "Seconds Running"(w403) -> ()
          n168 = local read "Exit"() -> (w404:bool)
          n169 = Greater Or Equal?(x=w403, y=w408) -> (x >= y?=w406:bool)
          n170 = Or(x=w406, y=w404) -> (x .or. y?=w405:bool)
        }
        n171 = call <vilib>:"Add State(s) to Queue__JKI_lib_State_Machine.vi"("State(s) in (\"\")"=w402) -> ("States Out"=w401:string)  [unwired: 14 in]
      }
    }
  }
